vi "Evaluate Status.vi"(11 "Statuses":T1[](array[typedef])) -> (3 "Status":T1=enum."Passed")   [LabVIEW 2020, in "Result Model.lvclass"]
uses:
  Result Model.lvclass
  Core/Result/Status.ctl
  Core/Result/Result.lvlib
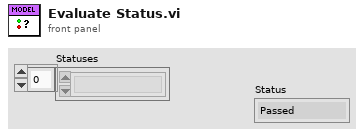
[diagram p1: front panel]
types:
  T1 = typedef "Result.lvlib/Status.ctl" = enum16{"", "Passed", "Failed", "Error", "Skipped", "Setup Error", "Broken", "Teardown Error"}
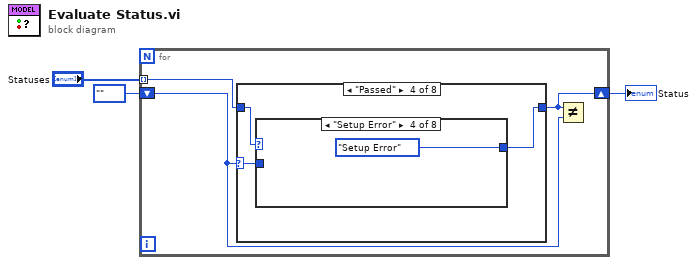
[diagram p0: block diagram]
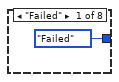
[diagram p3: hidden frame]
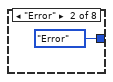
[diagram p4: hidden frame]
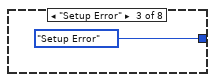
[diagram p5: hidden frame]
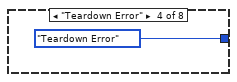
[diagram p6: hidden frame]
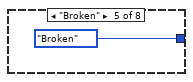
[diagram p7: hidden frame]
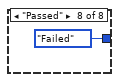
[diagram p9: hidden frame]
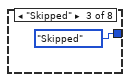
[diagram p11: hidden frame]
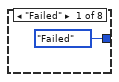
[diagram p12: hidden frame]
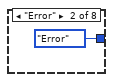
[diagram p13: hidden frame]
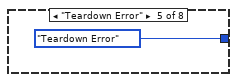
[diagram p15: hidden frame]
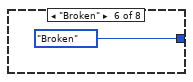
[diagram p16: hidden frame]
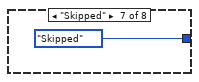
[diagram p17: hidden frame]
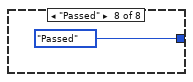
[diagram p18: hidden frame]
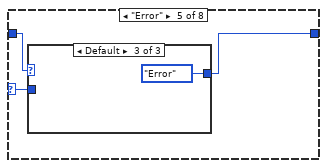
[diagram p19: hidden frame]
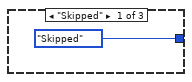
[diagram p20: hidden frame]
diagram:
  n1 = for {
    tunnel: "Statuses" -> [w4] mode=indexing
    shift-right: [w5] -> w2
    shift-left: Status."" ("Current") -> [w6]
    n2 = case shown="\"Passed\"" w6 {
      selector: w6 -> [w7 _ _ w20 w31 _ _ _]
      tunnel: w4 -> [w9 w18 _ w22 w32 w37 w41 w45]
      tunnel: [w8 w18 Status."Skipped" ("Merged Status") w21 w33 w38 w42 w46] -> w5
      frame "Failed" {
        n3 = case shown="\"\"" w9 {
          tunnel: [Status."Failed" ("Merged Status") Status."Error" ("Merged Status") Status."Setup Error" ("Merged Status") Status."Teardown Error" ("Merged Status") Status."Broken" ("Merged Status") w15 w16 Status."Failed" ("Merged Status")] -> w8
          tunnel: w7 -> [_ _ _ _ _ w15 w16 _]
          frame "Failed" {
          }
          frame "Error" {
          }
          frame "Setup Error" {
          }
          frame "Teardown Error" {
          }
          frame "Broken" {
          }
          frame "" {
          }
          frame "Skipped" {
          }
          frame "Passed" {
          }
        }
      }
      frame "" {
      }
      frame "Skipped" {
      }
      frame "Passed" {
        n4 = case shown="\"Setup Error\"" w22 {
          tunnel: [Status."Failed" ("Merged Status") Status."Error" ("Merged Status") w25 Status."Setup Error" ("Merged Status") Status."Teardown Error" ("Merged Status") Status."Broken" ("Merged Status") Status."Skipped" ("Merged Status") Status."Passed" ("Merged Status")] -> w21
          tunnel: w20 -> [_ _ w25 _ _ _ _ _]
          frame "Failed" {
          }
          frame "Error" {
          }
          frame "" {
          }
          frame "Setup Error" {
          }
          frame "Teardown Error" {
          }
          frame "Broken" {
          }
          frame "Skipped" {
          }
          frame "Passed" {
          }
        }
      }
      frame "Error" {
        n5 = case shown="Default" w32 {
          tunnel: [Status."Skipped" ("Merged Status") w35 Status."Error" ("Merged Status")] -> w33
          tunnel: w31 -> [_ w35 _]
          frame "Skipped" {
          }
          frame "" {
          }
          frame Default {
          }
        }
      }
      frame "Setup Error" {
        n6 = case shown="Default" w37 {
          tunnel: [Status."Skipped" ("Merged Status") Status."Setup Error" ("Merged Status")] -> w38
          frame "Skipped" {
          }
          frame Default {
          }
        }
      }
      frame "Broken" {
        n7 = case shown="Default" w41 {
          tunnel: [Status."Broken" ("Merged Status") Status."Setup Error" ("Merged Status")] -> w42
          frame Default {
          }
          frame "Setup Error" {
          }
        }
      }
      frame "Teardown Error" {
        n8 = case shown="Default" w45 {
          tunnel: [Status."Skipped" ("Merged Status") Status."Teardown Error" ("Merged Status")] -> w46
          frame "Skipped" {
          }
          frame Default {
          }
        }
      }
    }
    n9 = Not Equal?(x=w5, y=w6) -> ()  [unwired: 1 out]
  }
  "Status" <- w2
